vi "getStrain.vi"(6 "Channel":i32, 8 "error in (no error)":errorcluster, 11 "Instrument.Strain in":refnum<class "Instrument.Strain.lvclass">) -> (0 "error out":errorcluster, 2 "Strain (V)":dbl, 3 "Instrument.Strain out":refnum<class "Instrument.Strain.lvclass">)   [LabVIEW 2019, in "Instrument.Strain.lvclass"]
uses:
  Instrument.Strain.lvclass
  Typedefs/Strain.Commands--Enum.ctl
  b7c9f357-29aa-4e5f-be24-c57abdc517bc.vi
  b7c9f357-29aa-4e5f-be24-c57abdc517bc.vi/d53ee88d-cc6e-4e5d-a09e-c74db25cf8bf.vi
  b7c9f357-29aa-4e5f-be24-c57abdc517bc.vi/d2c209c6-58c4-4e27-b6e9-cc8ef8a93957.vi
  <vilib>/Utility/Data Type/Get Type Information.vi
  <vilib>/JDP Science/JSONtext/JSON text to Variant.vi
  <vilib>/JDP Science/JSONtext/LVClass Serializer/JSONtext LVClass Serializer.lvclass
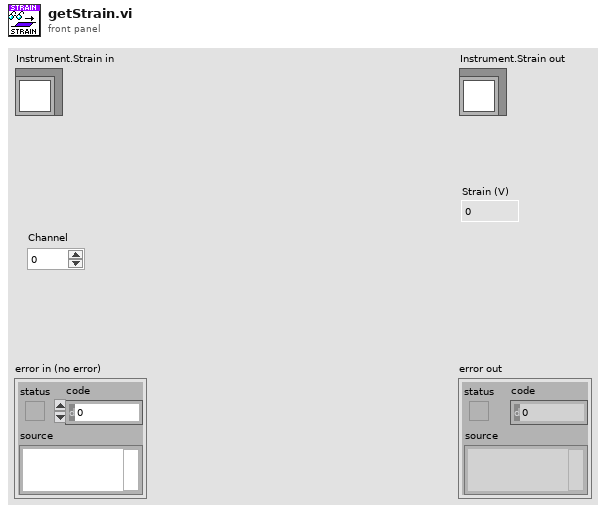
[diagram p1: front panel]
types:
  T1 = typedef "Instrument.Strain.lvclass/Strain.Commands--Enum.ctl" = enum16{"getStrain", "setStrain"}
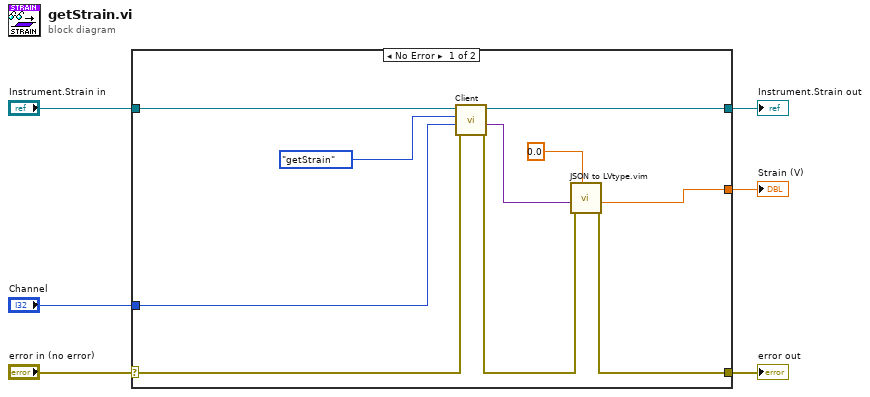
[diagram p0: block diagram]
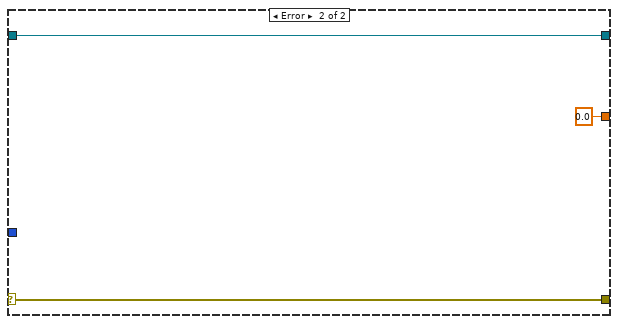
[diagram p2: hidden frame]
diagram:
  n1 = case shown="No Error" "error in (no error)" {
    selector: "error in (no error)" -> [w12 w19]
    tunnel: [w7 w19] -> w5
    tunnel: [w15 w18] -> w3
    tunnel: "Instrument.Strain in" -> [w13 w18]
    tunnel: "Channel" -> [w16 _]
    tunnel: [w11 0.0 ("Data out")] -> w1
    frame No Error {
      n2 = call-dynamic "Client.vi"("error in (no error)"=w12, "Data in"=w16, "Command in"=Strain.Commands--Enum."getStrain" ("Command"), "Instrument in"=w13) -> ("error out"=w8:errorcluster, "Data out"=w9:variant, "Instrument out"=w15:refnum<class "Instrument.Strain.lvclass">)  [unwired: 4 in, 1 out]
      n3 = call "JSON to LVtype.vim"("type"=0.0, "error in (no error)"=w8, "JSON Data in"=w9) -> ("error out"=w7:errorcluster, "Data out"=w11:dbl)  [unwired: 7 in]
    }
    frame Error {
    }
  }
  "error out" <- w5
  "Instrument.Strain out" <- w3
  "Strain (V)" <- w1
